vi "Main.vi"(11 "Module Admin":refnum<class "Delacor_lib_QMH_Cloneable Module Admin.lvclass">) -> ()   [LabVIEW 2019, in "Mensajes.lvlib"]
doc: "This template is based off of the Queued Message Handler design pattern and the Queued Message Handler project template that ships with LabVIEW.\n\nThe main difference is that the queue is private to this module and communication between modules is performed via Broadcast and Request events.\n\nRequest events are wrapped in public API methods and are handled in the Event Handling Loop (EHL) of this VI. Any module can register for Broadcast events sent by this module. The EHL generates messages based on user interface actions.\n\nThe Message Handling Loop (MHL) processes messages generated by the EHL, or by other messages. The messages are string values, so new messages can be added easily to the Message Cases case structure in the MHL. Each message cluster can also provide an optional value for Message Data, which is a variant that can be converted to whatever message-specific data is required.\n_____\nBased on DQMH Dev Tools: Project Template 7.1.0.1503."
uses:
  Mensajes.lvlib
  <vilib>/Delacor/Delacor QMH/Libraries/Cloneable Module Admin_class/Delacor_lib_QMH_Cloneable Module Admin.lvclass
  C:/Program Files (x86)/National Instruments/LabVIEW 2024/vi.lib/Delacor/Delacor QMH/Libraries/Module Admin_class/Delacor_lib_QMH_Module Admin.lvclass
  Module Data--cluster.ctl
  <vilib>/Delacor/Delacor QMH/Libraries/Cloneable Module Admin_class/Delacor_lib_QMH_Cloneable Module Admin.lvclass/Delacor_lib_QMH_Cloneable Module Admin.ctl
  Stop Argument--cluster.ctl
  <vilib>/Delacor/Delacor QMH/Libraries/Message Queue_class/Delacor_lib_QMH_Message Queue.lvclass/Delacor_lib_QMH_Message Queue.ctl
  <vilib>/Delacor/Delacor QMH/Libraries/Module Admin_class/Delacor_lib_QMH_Module Admin.lvclass/Delacor_lib_QMH_Module Admin.ctl
  Draw FP in Subpanel Argument--cluster.ctl
  Remove From Subpanel Argument--cluster.ctl
  Display Message Argument--cluster.ctl
  Set Display Style Argument--cluster.ctl
  <vilib>/Utility/miscctls.llb/LVPointTypeDef.ctl
  <vilib>/Delacor/Delacor QMH/Libraries/Cloneable Module Admin_class/Delacor_lib_QMH_Get Module ID.vi
  <vilib>/Delacor/Delacor QMH/Libraries/Message Queue_class/Delacor_lib_QMH_Enqueue Message (Single).vi
  <vilib>/Delacor/Delacor QMH/Libraries/Module Admin_class/Delacor_lib_QMH_Get External Launch.vi
  <vilib>/Delacor/Delacor QMH/Libraries/Message Queue_class/Delacor_lib_QMH_Message Queue.lvclass
panel:
  out "Message":string
  out "error out":errorcluster
  out "Status":string
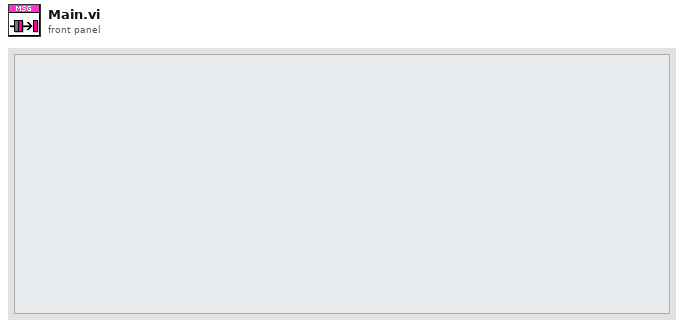
[diagram p1: front panel]
types:
  T1 = typedef "Mensajes.lvlib/Request Events--cluster.ctl" = cluster{"Stop Module":refnum<user-event>, "Show Panel":refnum<user-event>, "Hide Panel":refnum<user-event>, "Show Diagram":refnum<user-event>, "Get Module Execution Status":refnum<user-event>, "Draw FP in Subpanel":refnum<user-event>, "Remove From Subpanel":refnum<user-event>, "Display Message":refnum<user-event>, "Set Display Style":refnum<user-event>}
  T2 = typedef "Mensajes.lvlib/Module Data--cluster.ctl" = cluster{"Status":string, "Sub Panel":refnum<vi>, "Message Ref":refnum<vi>}
  T3 = enum32{"invalid lock state", "Not Locked", "Locked (No Password)", "Password-protected"}
  T4 = typedef "Mensajes.lvlib/Stop Argument--cluster.ctl" = cluster{"Module ID":i32, "Origin":string, "Exit via Stop Module Req?":bool, "Wait for Module to stop?":bool}
  T5 = typedef "Mensajes.lvlib/Draw FP in Subpanel Argument--cluster.ctl" = cluster{"Module ID":i32, "Sub Panel":refnum<vi>}
  T6 = typedef "Mensajes.lvlib/Remove From Subpanel Argument--cluster.ctl" = cluster{"Module ID":i32, "Boolean":bool}
  T7 = typedef "Mensajes.lvlib/Display Message Argument--cluster.ctl" = cluster{"Module ID":i32, "Message":string}
  T8 = typedef "Mensajes.lvlib/Set Display Style Argument--cluster.ctl" = cluster{"Module ID":i32, "Display Style":enum16{"Normal", "Backslash", "Password", "Hexadecimal"}}
  T9 = enum16{"Normal", "Backslash", "Password", "Hexadecimal"}
  T10 = typedef "LVPointTypeDef.ctl" = cluster{"Horizontal":i16, "Vertical":i16}
  T11 = enum32{"Invalid", "Standard", "Closed", "Hidden", "Minimized", "Maximized"}
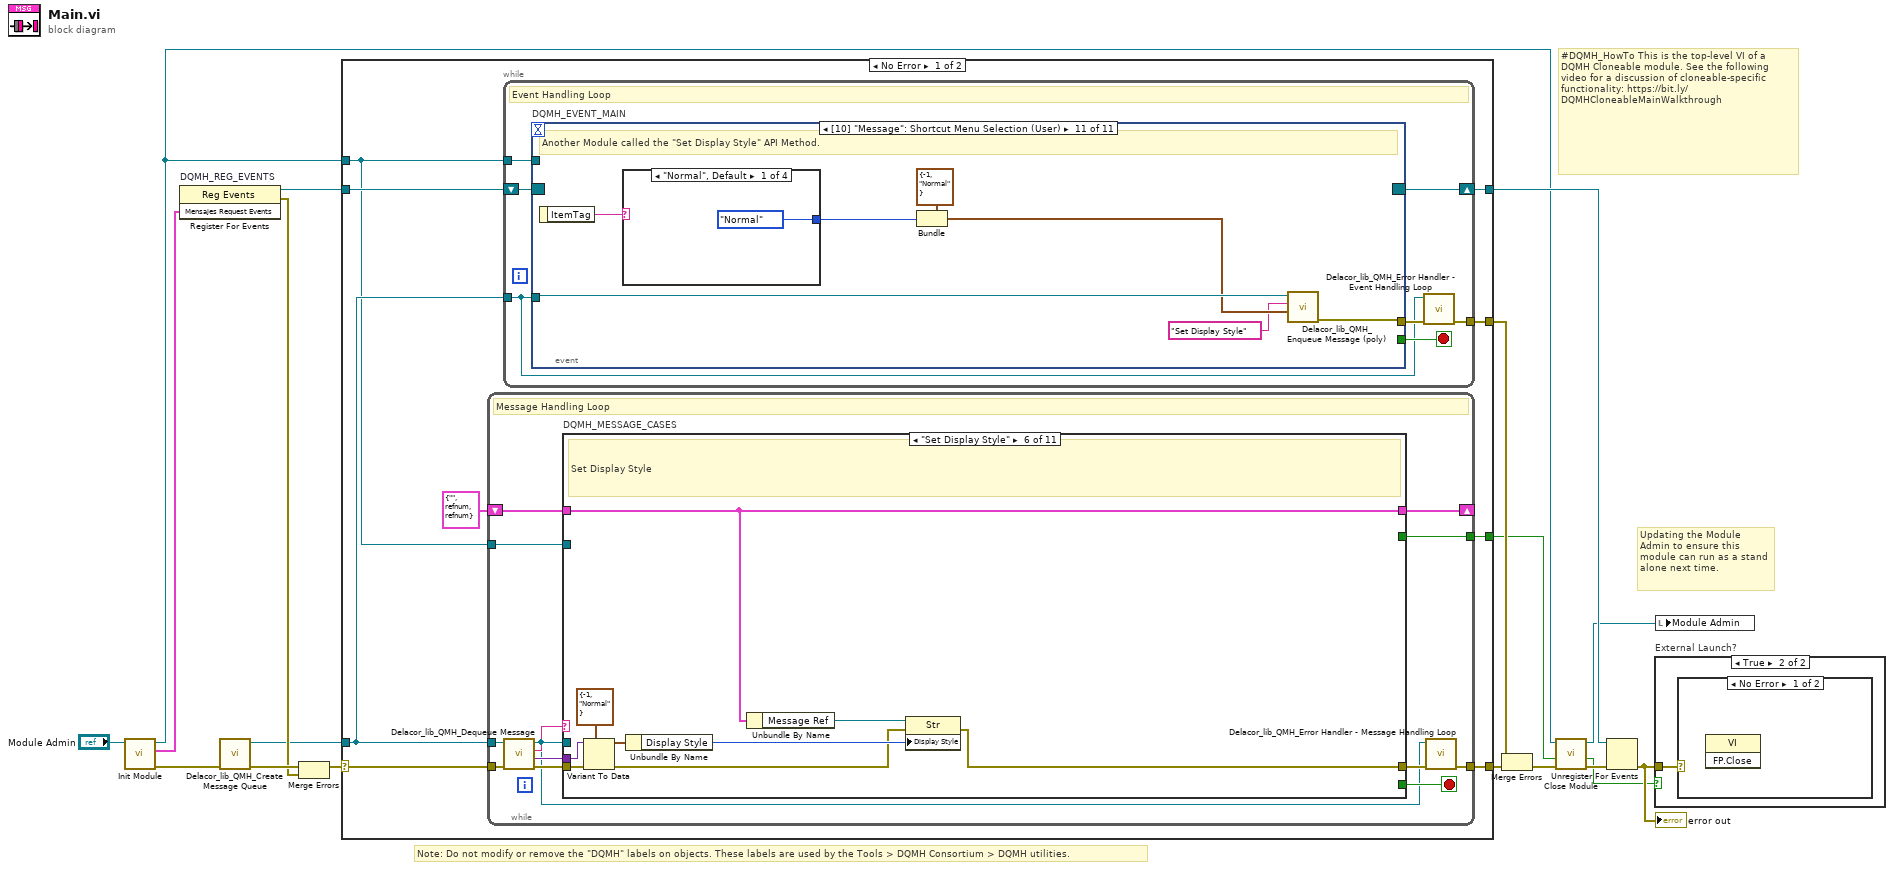
[diagram p0: block diagram]
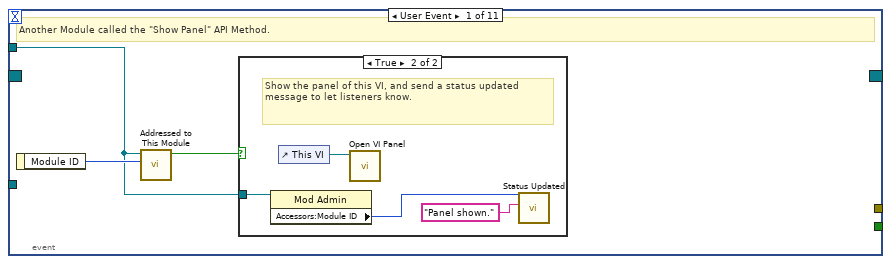
[diagram p2: hidden frame]
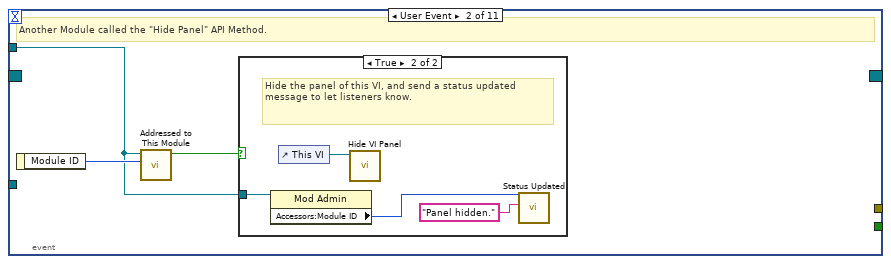
[diagram p4: hidden frame]
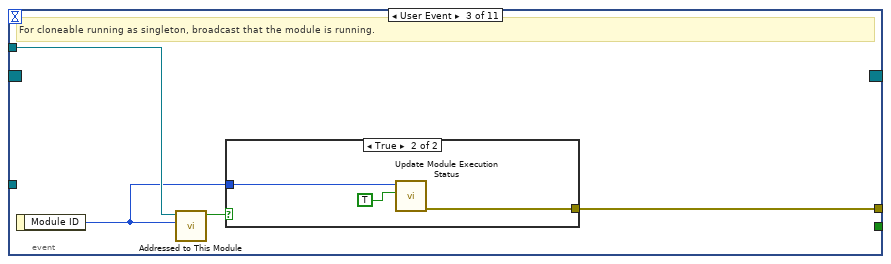
[diagram p6: hidden frame]
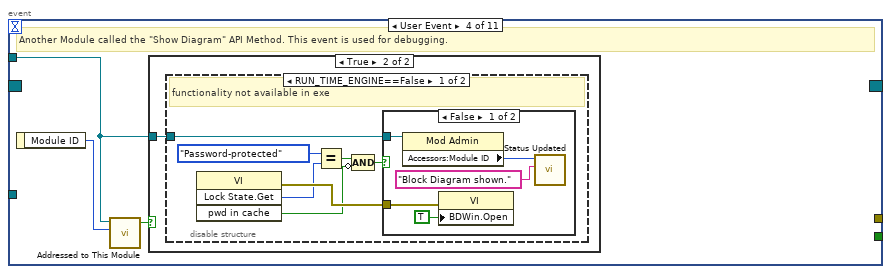
[diagram p8: hidden frame]
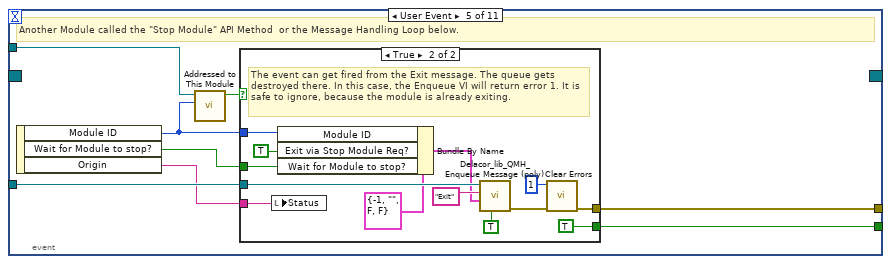
[diagram p12: hidden frame]
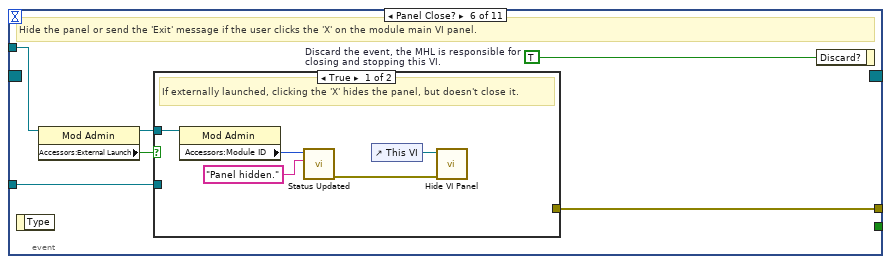
[diagram p14: hidden frame]
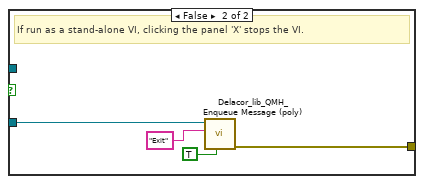
[diagram p15: hidden frame]
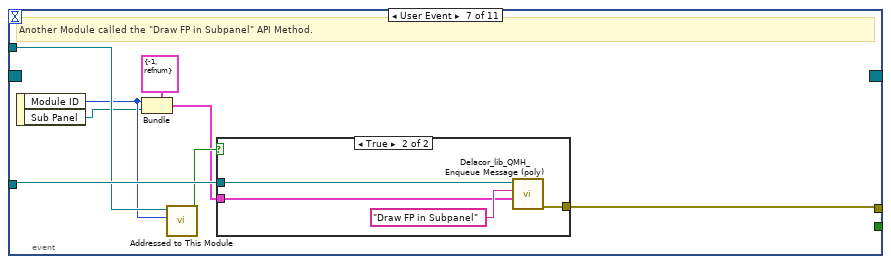
[diagram p16: hidden frame]
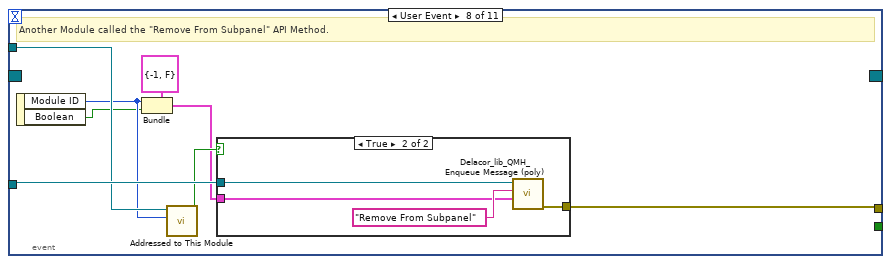
[diagram p18: hidden frame]
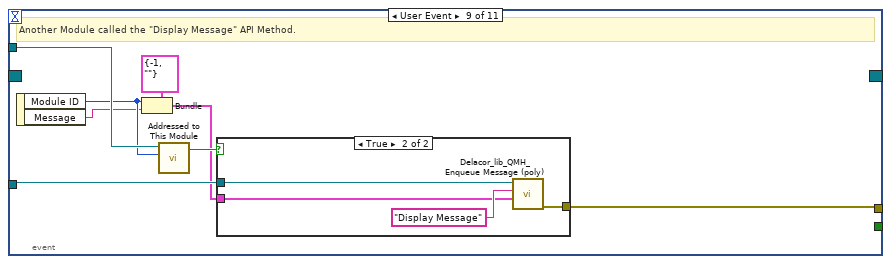
[diagram p20: hidden frame]
diagram:
  # "#DQMH_HowTo This is the top-level VI of a DQMH Cloneable module. See the following video for a discussion of cloneable-specific functionality: https://bit.ly/DQMHCloneableMainWalkthrough"
  # "Note: Do not modify or remove the \"DQMH\" labels on objects. These labels are used by the Tools > DQMH Consortium > DQMH utilities."
  # "Updating the Module Admin to ensure this module can run as a stand alone next time."
  n1 = call "Init Module.vi"("Cloneable Module Admin in"="Module Admin") -> ("error out"=w15:errorcluster, "Mensajes Request Events"=w7:T1, "Cloneable Module Admin out"=w4:refnum<class "Delacor_lib_QMH_Cloneable Module Admin.lvclass">)  [unwired: 8 in]
  n2 = register-events "DQMH_REG_EVENTS"(w7) -> (reference out=w8:refnum<event-registration>, error out=w10:errorcluster)  [unwired: 2 in]
  n3 = call <vilib>:"Delacor_lib_QMH_Create Message Queue.vi"("error in"=w15) -> ("error out"=w12:errorcluster, "Message Queue"=w6:refnum<class "Delacor_lib_QMH_Message Queue.lvclass">)  [unwired: 9 in]
  n4 = Merge Errors(w12, w10) -> (w11:errorcluster)
  n5 = case shown="No Error" w11 {
    selector: w11 -> [w25 w329]
    tunnel: [w27 w328] -> w16
    tunnel: [w24 w327] -> w9
    tunnel: w8 -> [w22 w327]
    tunnel: w6 -> [w21 w320]
    tunnel: [w26 _] -> w17
    tunnel: w4 -> [w20 w323]
    tunnel: [w19 _] -> w2
    frame No Error {
      n6 = while {
        tunnel: w21 -> [w167]
        shift-right: [w174] -> _
        shift-left: T2 {"Status"="", "Sub Panel"=refnum, "Message Ref"=refnum} ("Data Cluster") -> [w175]
        tunnel: w25 -> [w178]
        tunnel: [w176] -> w27
        tunnel: w20 -> [w169]
        tunnel: [w168] -> w19
        stop <- w173 stop-if-true
        # "Message Handling Loop"
        n7 = call-dynamic "Delacor_lib_QMH_Dequeue Message.vi"("error in"=w178, "Message Queue in"=w167) -> ("error out"=w177:errorcluster, "Message Data"=w171:variant, "Message"=w172:string, "Message Queue out"=w170:refnum<class "Delacor_lib_QMH_Message Queue.lvclass">)  [unwired: 6 in]
        n8 = case "DQMH_MESSAGE_CASES" shown="\"Set Display Style\"" w172 {
          selector: w172 -> [_ _ _ _ _ _ _ _ _ _ w309]
          tunnel: w170 -> [_ _ _ _ _ _ _ _ w273 w301 _]
          tunnel: w177 -> [w199 w203 w222 w242 w257 w266 w269 w271 w283 w307 w318]
          tunnel: [w197 w203 w218 w240 w255 w258 w268 w271 w279 w302 w319] -> w179
          tunnel: w175 -> [w190 w202 w208 w234 w256 w262 w267 w270 w277 w291 w316]
          tunnel: [w189 w202 w209 w230 w256 w262 w267 w270 w277 w291 w316] -> w174
          tunnel: [_ _ _ _ _ _ _ _ _ w300 _] -> w173
          tunnel: w171 -> [_ _ w217 w239 w254 w265 _ _ w276 w298 _]
          tunnel: w169 -> [w185 _ w206 w233 w251 _ _ _ w275 w293 w315]
          tunnel: [_ _ _ _ _ _ _ _ _ w296 _] -> w168
          frame "Initialize" {
            w182 = "Initial Message" ("Initial Message")
            # "Initialize - Any operation that needs to be done before the module can receive messages. Synchronize Caller Events.vi will inform Start Module.vi that the module has launched and is ready to receive messages. Module Did Init.vi will broadcast that the module initialized."
            n9 = call "Synchronize Caller Events.vi"("error in"=w199, "Module Admin"=w185) -> ("error out"=w198:errorcluster, "Module Admin out"=w184:refnum<class "Delacor_lib_QMH_Cloneable Module Admin.lvclass">)  [unwired: 8 in]
            n10 = property on="Property Node" class="Mod Admin"(reference=w184) -> ("Accessors:Module ID"=w181:i32, "Accessors:External Launch"=w186:bool)  [unwired: 1 in, 2 out]
            n11 = call "Module Name--constant.vi"("Module ID"=w181) -> ("Module Name"=w194:string)  [unwired: 10 in]
            n12 = property on="Property Node" class="VI"("Front Panel.Title"=w194) -> (reference out=w196:refnum<vi>, error out=w201:errorcluster)  [unwired: 2 in]
            n13 = Select(t=T11."Hidden" ("State"), s=w186, f=T11."Standard" ("State")) -> (s? t:f=w191:T11)
            n14 = control-ref of="Message"() -> (w180:refnum<vi>)
            n15 = invoke on="Invoke Node" class="VI" method="FP.Open"(reference=w196, error in=w201, "State"=w191) -> (reference out=w195:refnum<vi>, error out=w200:errorcluster)  [unwired: 2 in, 3 out]
            n16 = Bundle By Name(cluster=w190, "Message Ref"=w180, "Status"=w182) -> (w189:T2)
            n17 = invoke on="Invoke Node" class="VI" method="FP.Center"(reference=w195, error in=w200) -> ()  [unwired: 1 in, 3 out]
            n18 = property on="Pane" class="Pane"("Origin"=T10 {"Horizontal"=0, "Vertical"=0}) -> ()  [unwired: 2 in, 2 out]
            n19 = call "Module Name--constant.vi"("Module ID"=w181) -> ("Module Name"=w187:string)  [unwired: 10 in]
            n20 = call "Module Did Init.vi"("error in"=w198, "Initialized?"=TRUE, "Origin"=w187, "Module ID"=w181) -> ("error out"=w197:errorcluster)  [unwired: 7 in]
            "Status" <- w182
          }
          frame "---Module Specific---" {
            # "Separator -- The following cases handle messages specific to this Module."
          }
          frame "Draw FP in Subpanel" {
            # "Draw FP in Subpanel"
            n21 = Variant To Data(error in=w222, type=T5 {"Module ID"=-1, "Sub Panel"=refnum} ("Draw FP in Subpanel Argument"), Variant=w217) -> (data=w215:T5, error out=w219:errorcluster)
            n22 = property class="Mod Admin"(reference=w206) -> ("Accessors:Module ID"=w205:i32)  [unwired: 1 in, 2 out]
            n23 = Unbundle By Name(w215) -> ("Sub Panel"=w207:refnum<vi>)
            n24 = control-ref of="This VI"() -> (w212:refnum<vi>)
            n25 = property class="VI"(reference=w212, error in=w219) -> (reference out=w211:refnum<vi>, error out=w220:errorcluster, "FP.State"=w210:T11)
            n26 = case shown="\"Closed\"" w210 {
              tunnel: [w223 w226] -> w213
              tunnel: [w224 w228] -> w221
              tunnel: w220 -> [w224 w227]
              tunnel: w211 -> [w223 w225]
              frame "Closed" {
              }
              frame "Standard", Default {
                n27 = invoke class="VI" method="FP.Close"(reference=w225, error in=w227) -> (reference out=w226:refnum<vi>, error out=w228:errorcluster)  [unwired: 1 in, 1 out]
              }
            }
            n28 = invoke class="SubPnl" method="Insert VI"(reference=w207, error in=w221, "VI Ref"=w213) -> (reference out=w214:refnum<vi>, error out=w218:errorcluster)  [unwired: 1 in, 2 out]
            n29 = call "Status Updated.vi"("error in"=w218, "Status"="Front Panel Inserted in Subpanel", "Module ID"=w205) -> ()  [unwired: 8 in, 1 out]
            n30 = Bundle By Name(cluster=w208, "Sub Panel"=w214) -> (w209:T2)
          }
          frame "Remove From Subpanel" {
            # "Remove From Subpanel"
            n31 = Variant To Data(error in=w242, type=T6 {"Module ID"=-1, "Boolean"=FALSE} ("Remove From Subpanel Argument"), Variant=w239) -> (data=w237:T6, error out=w241:errorcluster)
            n32 = Unbundle By Name(w237) -> ()  [unwired: 2 out]
            n33 = property class="Mod Admin"(reference=w233) -> ("Accessors:Module ID"=w232:i32)  [unwired: 1 in, 2 out]
            n34 = Unbundle By Name(w234) -> ("Sub Panel"=w236:refnum<vi>)
            n35 = Not A Number/Path/Refnum?(number/path/refnum=w236) -> (NaN/Path/Refnum?=w235:bool)
            n36 = case shown="False" w235 {
              tunnel: w241 -> [w246 w248]
              tunnel: [w245 w248] -> w240
              tunnel: w236 -> [w244 _]
              tunnel: ["Panel Removed from Subpanel" "This module has not been inserted into the subpanel"] -> w231
              frame False {
                n37 = invoke class="SubPnl" method="Remove VI"(reference=w244, error in=w246) -> (error out=w245:errorcluster)  [unwired: 1 in, 2 out]
              }
              frame True {
              }
            }
            n38 = Bundle By Name(cluster=w234, "Sub Panel"=refnum<vi> refnum) -> (w230:T2)
            n39 = call "Status Updated.vi"("error in"=w240, "Status"=w231, "Module ID"=w232) -> ()  [unwired: 8 in, 1 out]
          }
          frame "Display Message" {
            # "Display Message"
            n40 = Variant To Data(error in=w257, type=T7 {"Module ID"=-1, "Message"=""} ("Display Message Argument"), Variant=w254) -> (data=w252:T7, error out=w255:errorcluster)
            n41 = property class="Mod Admin"(reference=w251) -> ("Accessors:Module ID"=w250:i32)  [unwired: 1 in, 2 out]
            n42 = Unbundle By Name(w252) -> ("Message"=w249:string)  [unwired: 1 out]
            "Message" <- w249
            n43 = call "Status Updated.vi"("Status"=w249, "Module ID"=w250) -> ()  [unwired: 9 in, 1 out]
          }
          frame "Set Display Style" {
            # "Set Display Style"
            n44 = Variant To Data(error in=w266, type=T8 {"Module ID"=-1, "Display Style"=enum."Normal"} ("Set Display Style Argument"), Variant=w265) -> (data=w263:T8, error out=w259:errorcluster)
            n45 = Unbundle By Name(w263) -> ("Display Style"=w260:T9)
            n46 = Unbundle By Name(w262) -> ("Message Ref"=w261:refnum<vi>)
            n47 = property class="Str"(reference=w261, error in=w259, "Display Style"=w260) -> (error out=w258:errorcluster)  [unwired: 1 out]
          }
          frame "---Copy This Frame---" {
            # "Duplicate this frame when creating new messages.  Change this comment in the duplicated frame to describe this message."
            n48 = Merge Errors(w269) -> (w268:errorcluster)
          }
          frame "---Exit and Error Handling---" {
            # "Separator - the following cases handle errors and exit messages."
          }
          frame "Error" {
            # "#DQMH_CodeRecommended - If the module is running in standalone mode (External Launch = FALSE), this code will pop up an error dialog and call the 'Exit' message if an error occurs. Add more fine-grained error management here."
            # "Error - Check the error message data and respond accordingly. This message is sent by the \"Error Handler\" VIs at the end of each loop in this application."
            n49 = property on="Property Node" class="Mod Admin"(reference=w275) -> ("Accessors:External Launch"=w274:bool, "Accessors:Module ID"=w272:i32)  [unwired: 1 in, 2 out]
            n50 = Variant To Data(error in=w283, type=errorcluster {"status"=FALSE, "code"=0, "source"=""} ("error constant"), Variant=w276) -> (data=w278:errorcluster, error out=w281:errorcluster)
            n51 = local write "error out"(w278) -> ()
            n52 = call "Error Reported.vi"("Error"=w278, "Module ID"=w272) -> ()  [unwired: 9 in, 1 out]
            n53 = case shown="False" w274 {
              tunnel: [w288 _] -> w280
              tunnel: w273 -> [w286 _]
              tunnel: w278 -> [w287 _]
              frame False {
                n54 = disable-structure shown="Default" {
                  disable-tunnel: w287 -> [w289 _]
                  frame condition #0 (active) {
                    # "If the module is running standalone, then pop up an error dialog and call the \"Exit\" message."
                    n55 = call <vilib>:"Simple Error Handler.vi"("error in (no error)"=w289) -> ()  [unwired: 4 in, 5 out]
                  }
                  frame condition #1 {
                    # "To prevent the Simple Error Handler VI from being loaded (e.g. when deploying to a Real-Time target), add the Conditional Disable Symbol \"DQMH_Disable_SEH\" to your project and set it to TRUE."
                  }
                }
                n56 = call-poly <vilib>:"Delacor_lib_QMH_Enqueue Message (poly).vi"("Priority Message? (F)"=TRUE, "Message"="Exit", "Message Queue in"=w286) -> ("error out"=w288:errorcluster)  [unwired: 7 in, 1 out]
              }
              frame True {
                # "If the module was launched externally, calling the Error Reported broadcast VI is the only action performed by the \"Error\" message. The module's caller can then process the error appropriately."
              }
            }
            n57 = Merge Errors(w281, w280) -> (w279:errorcluster)
          }
          frame "Exit" {
            w299 = 91  # 91: not all Exit messages will have an argument
            w300 = TRUE  # Stop the VI
            # "Release the message queue reference"
            # "#DQMH_CodeNeeded - Add any required cleanup code here."
            # "Exit - Exit the application."
            n58 = Variant To Data(error in=w307, type=T4 {"Module ID"=-1, "Origin"="", "Exit via Stop Module Req?"=FALSE, "Wait for Module to stop?"=FALSE} ("Stop Argument"), Variant=w298) -> (data=w295:T4, error out=w303:errorcluster)
            n59 = call <vilib>:"Clear Errors.vi"("error in (no error)"=w303, "specific error code to clear (0: all)"=w299) -> ("error out"=w306:errorcluster)  [unwired: 4 in, 1 out]
            n60 = property on="Property Node" class="Mod Admin"(reference=w293) -> ("Accessors:Module ID"=w292:i32)  [unwired: 1 in, 2 out]
            n61 = control-ref of="This VI"() -> (w294:refnum<vi>)
            n62 = call-dynamic "Delacor_lib_QMH_Release Message Queue.vi"("error in"=w306, "Message Queue"=w301) -> ("error out"=w305:errorcluster)  [unwired: 9 in]
            n63 = call "Handle Exit.vi"("Stop Argument"=w295, "Module Admin in"=w293, "VI reference"=w294) -> ("error out"=w304:errorcluster, "Wait for Stop?"=w296:bool)  [unwired: 7 in]
            n64 = Merge Errors(w305, w304) -> (w302:errorcluster)
            n65 = Unbundle By Name(w291) -> ("Sub Panel"=w290:refnum<vi>)
            n66 = call "Error Reported.vi"("Error"=w302, "Module ID"=w292) -> ()  [unwired: 9 in, 1 out]
            n67 = invoke class="SubPnl" method="Remove VI"(reference=w290) -> ()  [unwired: 2 in, 3 out]
          }
          frame Default {
            # "'Default' case only runs if there is a message that isn't defined in any of the other cases.  Output a programming error."
            n68 = property on="Property Node" class="Mod Admin"(reference=w315) -> ("Accessors:Module ID"=w314:i32)  [unwired: 1 in, 2 out]
            n69 = call "Module Name--constant.vi"("Module ID"=w314) -> ("Module Name"=w308:string)  [unwired: 10 in]
            n70 = Format Into String(format string="The invalid message string \"%s\" was received in the Message Handling Loop for module \"%s\".", w309, w308) -> (resulting string=w311:string)  [unwired: 2 in, 1 out]
            n71 = call <vilib>:"Error Cluster From Error Code.vi"("show call chain? (False)"=TRUE, "error message (\"\")"=w311, "error code (0)"=1) -> ("error out"=w317:errorcluster)  [unwired: 6 in]
            n72 = Merge Errors(w318, w317) -> (w319:errorcluster)
          }
        }
        n73 = call-dynamic "Delacor_lib_QMH_Error Handler - Message Handling Loop.vi"("error in"=w179, "Message Queue in"=w170) -> ("dup error in"=w176:errorcluster)  [unwired: 8 in, 1 out]
      }
      n74 = while {
        tunnel: w21 -> [w28]
        shift-right: [w31] -> w24
        shift-left: w22 -> [w32]
        tunnel: [w33] -> w26
        tunnel: w20 -> [w29]
        stop <- w30 stop-if-true
        # "Event Handling Loop"
        n75 = event "DQMH_EVENT_MAIN" shown="[10] \"Message\": Shortcut Menu Selection (User)" {
          selector: w32 -> [_ _ _ _ _ _ _ _ _ _ _]
          dyn-events: [_ _ _ _ _ _ _ _ _ _ _] -> w31
          timeout: _ -> [_ _ _ _ _ _ _ _ _ _ _]
          tunnel: [_ _ _ _ w75 _ _ _ _ _ _] -> w30
          tunnel: w28 -> [_ _ _ _ w78 w95 w114 w126 w139 w151 w162]
          tunnel: [_ _ w52 _ w79 w98 w115 w127 w132 w144 w159] -> w34
          tunnel: w29 -> [w35 w42 w50 w56 w77 w96 w112 w124 w137 w149 _]
          event User Event {
            # "Another Module called the \"Show Panel\" API Method."
            n76 = event-data() -> ("Module ID"=w36:i32)  [unwired: 1 in]
            n77 = call "Addressed to This Module.vi"("Module ID from Argument"=w36, "Module Admin"=w35) -> ("Addressed to this instance?"=w37:bool)  [unwired: 8 in, 1 out]
            n78 = case shown="True" w37 {
              tunnel: w35 -> [_ w39]
              frame False {
              }
              frame True {
                # "Show the panel of this VI, and send a status updated message to let listeners know."
                n79 = property on="Property Node" class="Mod Admin"(reference=w39) -> ("Accessors:Module ID"=w38:i32)  [unwired: 1 in, 2 out]
                n80 = control-ref of="This VI"() -> (w41:refnum<vi>)
                n81 = call "Open VI Panel.vi"("VI"=w41) -> ()  [unwired: 10 in, 1 out]
                n82 = call "Status Updated.vi"("Status"="Panel shown." ("format string"), "Module ID"=w38) -> ()  [unwired: 9 in, 1 out]
              }
            }
          }
          event User Event {
            # "Another Module called the \"Hide Panel\" API Method."
            n83 = event-data() -> ("Module ID"=w43:i32)  [unwired: 1 in]
            n84 = call "Addressed to This Module.vi"("Module ID from Argument"=w43, "Module Admin"=w42) -> ("Addressed to this instance?"=w44:bool)  [unwired: 8 in, 1 out]
            n85 = case shown="True" w44 {
              tunnel: w42 -> [_ w46]
              frame False {
              }
              frame True {
                # "Hide the panel of this VI, and send a status updated message to let listeners know."
                n86 = property on="Property Node" class="Mod Admin"(reference=w46) -> ("Accessors:Module ID"=w45:i32)  [unwired: 1 in, 2 out]
                n87 = control-ref of="This VI"() -> (w48:refnum<vi>)
                n88 = call "Hide VI Panel.vi"("VI"=w48) -> ()  [unwired: 10 in, 1 out]
                n89 = call "Status Updated.vi"("Status"="Panel hidden." ("format string"), "Module ID"=w45) -> ()  [unwired: 9 in, 1 out]
              }
            }
          }
          event User Event {
            # "For cloneable running as singleton, broadcast that the module is running."
            n90 = event-data() -> ("Module ID"=w49:i32)  [unwired: 1 in]
            n91 = call "Addressed to This Module.vi"("Module ID from Argument"=w49, "Module Admin"=w50) -> ("Addressed to this instance?"=w51:bool)  [unwired: 8 in, 1 out]
            n92 = case shown="True" w51 {
              tunnel: [_ w55] -> w52
              tunnel: w49 -> [_ w54]
              frame False {
              }
              frame True {
                n93 = call "Update Module Execution Status.vi"("Running?"=TRUE, "Module ID"=w54) -> ("error out"=w55:errorcluster)  [unwired: 9 in]
              }
            }
          }
          event User Event {
            # "Another Module called the \"Show Diagram\" API Method. This event is used for debugging."
            n94 = event-data() -> ("Module ID"=w57:i32)  [unwired: 1 in]
            n95 = call "Addressed to This Module.vi"("Module ID from Argument"=w57, "Module Admin"=w56) -> ("Addressed to this instance?"=w58:bool)  [unwired: 8 in, 1 out]
            n96 = case shown="True" w58 {
              tunnel: w56 -> [_ w59]
              frame False {
              }
              frame True {
                n97 = disable-structure shown="RUN_TIME_ENGINE==False" {
                  disable-tunnel: w59 -> [w60 _]
                  frame condition #0 (active) {
                    # "functionality not available in exe"
                    n98 = invoke on="Invoke Node" class="VI" method="Lock State.Get"() -> (error out=w66:errorcluster, "Get Lock State"=w65:T3, "pwd in cache"=w62:bool)  [unwired: 4 in, 1 out]
                    n99 = Equal?(x=T3."Password-protected", y=w65) -> (x = y?=w63:bool)
                    n100 = Compound Arithmetic op=AND(w63, invert w62) -> (w61:bool)
                    n101 = case shown="False" w61 {
                      tunnel: w66 -> [w71 _]
                      tunnel: w60 -> [w68 _]
                      frame False {
                        n102 = property on="Property Node" class="Mod Admin"(reference=w68) -> ("Accessors:Module ID"=w67:i32)  [unwired: 1 in, 2 out]
                        n103 = property on="Property Node" class="VI"(error in=w71, "BDWin.Open"=TRUE ("Block Diagram Window:Open")) -> ()  [unwired: 1 in, 2 out]
                        n104 = call "Status Updated.vi"("Status"="Block Diagram shown." ("format string"), "Module ID"=w67) -> ()  [unwired: 9 in, 1 out]
                      }
                      frame True {
                        # "Password-protected VI, and the password is not in the cache. Do not show the diagram."
                      }
                    }
                  }
                  frame condition #1 {
                  }
                }
              }
            }
          }
          event User Event {
            # "Another Module called the \"Stop Module\" API Method  or the Message Handling Loop below."
            n105 = event-data() -> ("Module ID"=w73:i32, "Wait for Module to stop?"=w74:bool, "Origin"=w72:string)  [unwired: 1 in]
            n106 = call "Addressed to This Module.vi"("Module ID from Argument"=w73, "Module Admin"=w77) -> ("Addressed to this instance?"=w76:bool)  [unwired: 8 in, 1 out]
            n107 = case shown="True" w76 {
              tunnel: [_ w91] -> w79
              tunnel: w78 -> [_ w87]
              tunnel: [_ TRUE] -> w75
              tunnel: w74 -> [_ w82]
              tunnel: w73 -> [_ w84]
              tunnel: w72 -> [_ w80]
              frame False {
              }
              frame True {
                # "The event can get fired from the Exit message. The queue gets destroyed there. In this case, the Enqueue VI will return error 1. It is safe to ignore, because the module is already exiting."
                n108 = local write "Status"(w80) -> ()
                n109 = Bundle By Name(cluster=T4 {"Module ID"=-1, "Origin"="", "Exit via Stop Module Req?"=FALSE, "Wait for Module to stop?"=FALSE} ("Stop Argument"), "Module ID"=w84, "Exit via Stop Module Req?"=TRUE, "Wait for Module to stop?"=w82) -> (w81:T4)
                n110 = call-poly <vilib>:"Delacor_lib_QMH_Enqueue Message (poly).vi"("Priority Message? (F)"=TRUE, "Message Data"=w81, "Message"="Exit", "Message Queue in"=w87) -> ("error out"=w92:errorcluster)  [unwired: 6 in, 1 out]
                n111 = call <vilib>:"Clear Errors.vi"("error in (no error)"=w92, "specific error code to clear (0: all)"=1) -> ("error out"=w91:errorcluster)  [unwired: 4 in, 1 out]
              }
            }
          }
          event Panel Close? {
            w97 = TRUE  # Discard the event, the MHL is responsible for closing and stopping this VI.
            # "Hide the panel or send the 'Exit' message if the user clicks the 'X' on the module main VI panel."
            n112 = event-data() -> ()  [unwired: 1 in, 1 out]
            n113 = property on="Property Node" class="Mod Admin"(reference=w96) -> (reference out=w93:refnum<class "Delacor_lib_QMH_Cloneable Module Admin.lvclass">, "Accessors:External Launch"=w94:bool)  [unwired: 1 in, 1 out]
            n114 = case shown="True" w94 {
              tunnel: w95 -> [_ w106]
              tunnel: [_ w107] -> w98
              tunnel: w93 -> [w100 _]
              frame True {
                # "If externally launched, clicking the 'X' hides the panel, but doesn't close it."
                n115 = property on="Property Node" class="Mod Admin"(reference=w100) -> ("Accessors:Module ID"=w99:i32)  [unwired: 1 in, 2 out]
                n116 = call "Status Updated.vi"("Status"="Panel hidden." ("format string"), "Module ID"=w99) -> ("error out"=w103:errorcluster)  [unwired: 9 in]
                n117 = control-ref of="This VI"() -> (w102:refnum<vi>)
                n118 = call "Hide VI Panel.vi"("error in"=w103, "VI"=w102) -> ()  [unwired: 9 in, 1 out]
              }
              frame False {
                # "If run as a stand-alone VI, clicking the panel 'X' stops the VI."
                n119 = call-poly <vilib>:"Delacor_lib_QMH_Enqueue Message (poly).vi"("Priority Message? (F)"=TRUE, "Message"="Exit", "Message Queue in"=w106) -> ("error out"=w107:errorcluster)  [unwired: 7 in, 1 out]
              }
            }
            n120 = event-data ("Event Filter Node")("Discard?"=w97) -> ()  [unwired: 1 in, 1 out]
          }
          event User Event {
            # "Another Module called the \"Draw FP in Subpanel\" API Method."
            n121 = event-data() -> ("Module ID"=w109:i32, "Sub Panel"=w108:refnum<vi>)  [unwired: 1 in]
            n122 = Bundle(cluster=T5 {"Module ID"=-1, "Sub Panel"=refnum} ("Draw FP in Subpanel Argument"), "Module ID"=w109, "Sub Panel"=w108) -> (w110:T5)
            n123 = call "Addressed to This Module.vi"("Module ID from Argument"=w109, "Module Admin"=w112) -> ("Addressed to this instance?"=w113:bool)  [unwired: 8 in, 1 out]
            n124 = case shown="True" w113 {
              tunnel: w114 -> [_ w118]
              tunnel: w110 -> [_ w116]
              tunnel: [_ w119] -> w115
              frame False {
              }
              frame True {
                n125 = call-poly <vilib>:"Delacor_lib_QMH_Enqueue Message (poly).vi"("Message Data"=w116, "Message"="Draw FP in Subpanel", "Message Queue in"=w118) -> ("error out"=w119:errorcluster)  [unwired: 7 in, 1 out]
              }
            }
          }
          event User Event {
            # "Another Module called the \"Remove From Subpanel\" API Method."
            n126 = event-data() -> ("Module ID"=w121:i32, "Boolean"=w120:bool)  [unwired: 1 in]
            n127 = Bundle(cluster=T6 {"Module ID"=-1, "Boolean"=FALSE} ("Remove From Subpanel Argument"), "Module ID"=w121, "Boolean"=w120) -> (w122:T6)
            n128 = call "Addressed to This Module.vi"("Module ID from Argument"=w121, "Module Admin"=w124) -> ("Addressed to this instance?"=w125:bool)  [unwired: 8 in, 1 out]
            n129 = case shown="True" w125 {
              tunnel: w126 -> [_ w130]
              tunnel: w122 -> [_ w128]
              tunnel: [_ w131] -> w127
              frame False {
              }
              frame True {
                n130 = call-poly <vilib>:"Delacor_lib_QMH_Enqueue Message (poly).vi"("Message Data"=w128, "Message"="Remove From Subpanel", "Message Queue in"=w130) -> ("error out"=w131:errorcluster)  [unwired: 7 in, 1 out]
              }
            }
          }
          event User Event {
            # "Another Module called the \"Display Message\" API Method."
            n131 = event-data() -> ("Module ID"=w134:i32, "Message"=w133:string)  [unwired: 1 in]
            n132 = Bundle(cluster=T7 {"Module ID"=-1, "Message"=""} ("Display Message Argument"), "Module ID"=w134, "Message"=w133) -> (w135:T7)
            n133 = call "Addressed to This Module.vi"("Module ID from Argument"=w134, "Module Admin"=w137) -> ("Addressed to this instance?"=w138:bool)  [unwired: 8 in, 1 out]
            n134 = case shown="True" w138 {
              tunnel: w139 -> [_ w143]
              tunnel: w135 -> [_ w141]
              tunnel: [_ w140] -> w132
              frame False {
              }
              frame True {
                n135 = call-poly <vilib>:"Delacor_lib_QMH_Enqueue Message (poly).vi"("Message Data"=w141, "Message"="Display Message", "Message Queue in"=w143) -> ("error out"=w140:errorcluster)  [unwired: 7 in, 1 out]
              }
            }
          }
          event User Event {
            # "Another Module called the \"Set Display Style\" API Method."
            n136 = event-data() -> ("Module ID"=w146:i32, "Display Style"=w145:T9)  [unwired: 1 in]
            n137 = Bundle(cluster=T8 {"Module ID"=-1, "Display Style"=enum."Normal"} ("Set Display Style Argument"), "Module ID"=w146, "Display Style"=w145) -> (w147:T8)
            n138 = call "Addressed to This Module.vi"("Module ID from Argument"=w146, "Module Admin"=w149) -> ("Addressed to this instance?"=w150:bool)  [unwired: 8 in, 1 out]
            n139 = case shown="True" w150 {
              tunnel: w151 -> [_ w155]
              tunnel: w147 -> [_ w153]
              tunnel: [_ w152] -> w144
              frame False {
              }
              frame True {
                n140 = call-poly <vilib>:"Delacor_lib_QMH_Enqueue Message (poly).vi"("Message Data"=w153, "Message"="Set Display Style", "Message Queue in"=w155) -> ("error out"=w152:errorcluster)  [unwired: 7 in, 1 out]
              }
            }
          }
          event "Message": Shortcut Menu Selection (User) {
            # "Another Module called the \"Set Display Style\" API Method."
            n141 = event-data() -> ("ItemTag"=w157:string)  [unwired: 1 in]
            n142 = case shown="\"Normal\", Default" w157 {
              tunnel: [T9."Normal" ("Display Style") T9."Backslash" ("Display Style") T9."Password" ("Display Style") T9."Hexadecimal" ("Display Style")] -> w156
              frame "Normal", Default {
              }
              frame "Backslash" {
              }
              frame "Password" {
              }
              frame "Hexadecimal" {
              }
            }
            n143 = Bundle(cluster=T8 {"Module ID"=-1, "Display Style"=enum."Normal"} ("Set Display Style Argument"), "Display Style"=w156) -> (w160:T8)  [unwired: 1 in]
            n144 = call-poly <vilib>:"Delacor_lib_QMH_Enqueue Message (poly).vi"("Message Data"=w160, "Message"="Set Display Style", "Message Queue in"=w162) -> ("error out"=w159:errorcluster)  [unwired: 7 in, 1 out]
          }
        }
        n145 = call-dynamic "Delacor_lib_QMH_Error Handler - Event Handling Loop.vi"("error in"=w34, "Message Queue in"=w28) -> ("dup error in"=w33:errorcluster)  [unwired: 8 in, 1 out]
      }
    }
    frame Error {
      n146 = call "Synchronize Caller Events.vi"("Module Admin"=w323) -> ("Module Admin out"=w322:refnum<class "Delacor_lib_QMH_Cloneable Module Admin.lvclass">)  [unwired: 9 in, 1 out]
      n147 = property on="Property Node" class="Mod Admin"(reference=w322) -> ("Accessors:Module ID"=w321:i32)  [unwired: 1 in, 2 out]
      n148 = call-dynamic "Delacor_lib_QMH_Release Message Queue.vi"("error in"=w329, "Message Queue"=w320) -> ("error out"=w328:errorcluster)  [unwired: 9 in]
      n149 = call "Module Name--constant.vi"("Module ID"=w321) -> ("Module Name"=w326:string)  [unwired: 10 in]
      n150 = Format Into String(format string="An error occurred during initialization. %s is no longer running.", w326) -> (resulting string=w324:string)  [unwired: 2 in, 1 out]
      n151 = call "Error Reported.vi"("Additional Information"=w324, "Error"=w328, "Module ID"=w321) -> ()  [unwired: 8 in, 1 out]
    }
  }
  n152 = Merge Errors(w17, w16) -> (w18:errorcluster)
  n153 = call "Close Module.vi"("error in"=w18, "Wait for stop?"=w2, "Module Admin in"=w4) -> ("error out"=w14:errorcluster, "External Launch"=w1:bool, "Module Admin out"=w3:refnum<class "Delacor_lib_QMH_Cloneable Module Admin.lvclass">)  [unwired: 6 in]
  n154 = Unregister For Events(event registration refnum=w9, error in=w14) -> (error out=w13:errorcluster)
  "error out" <- w13
  n155 = case "External Launch?" shown="True" w1 {
    tunnel: w13 -> [_ w330]
    frame False {
    }
    frame True {
      n156 = case shown="No Error" w330 {
        frame No Error {
          n157 = invoke class="VI" method="FP.Close"() -> ()  [unwired: 3 in, 3 out]
        }
        frame Error {
          n158 = disable-structure shown="Default" {
            frame condition #0 (active) {
              n159 = invoke class="VI" method="FP.Open"("Activate"=TRUE ("Activate?")) -> ()  [unwired: 4 in, 5 out]
            }
            frame condition #1 {
              # "Don't show panel on error if running inside a built EXE."
            }
          }
        }
      }
    }
  }
  n160 = local write "Module Admin"(w3) -> ()
